vi "Write Data.vi"(8 "error in (no error)":errorcluster, 9 "Publication Time":timestamp, 10 "Value":variant, 11 "TerminalValueBinding In":refnum<class "TerminalValueBinding.lvclass">) -> (0 "error out":errorcluster, 3 "TerminalValueBinding Out":refnum<class "TerminalValueBinding.lvclass">)   [LabVIEW 2017, in "TerminalValueBinding.lvclass"]
doc: "<License>\nCopyright © 2017 Composed Systems, LLC | All rights reserved\nwww.composed.io\n\nAuthor: Ethan Stern <ethan.stern@composed.io>\n\nThis software is provided \"AS IS\" WITHOUT WARRANTIES, either express or implied, AND IS FOR EDUCATIONAL PURPOSES ONLY.\n</License>"
uses:
  <vilib>/gpm_packages/@cs/transport/Source/Concrete/TerminalValueBinding/TerminalValueBinding.lvclass
  <vilib>/gpm_packages/@cs/transport/Source/Concrete/TerminalValueBinding/TerminalValueBinding.lvclass/TerminalValueBinding.ctl
  <vilib>/Utility/error.llb/Error Cluster From Error Code.vi
  <vilib>/ErrorRing/Error Ring.xnode
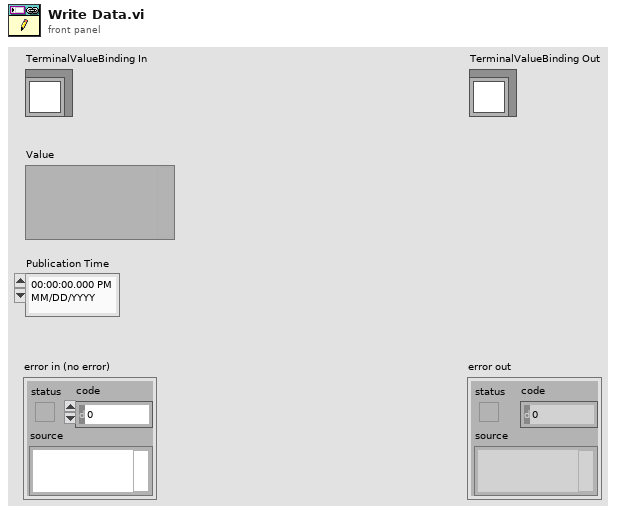
[diagram p1: front panel]
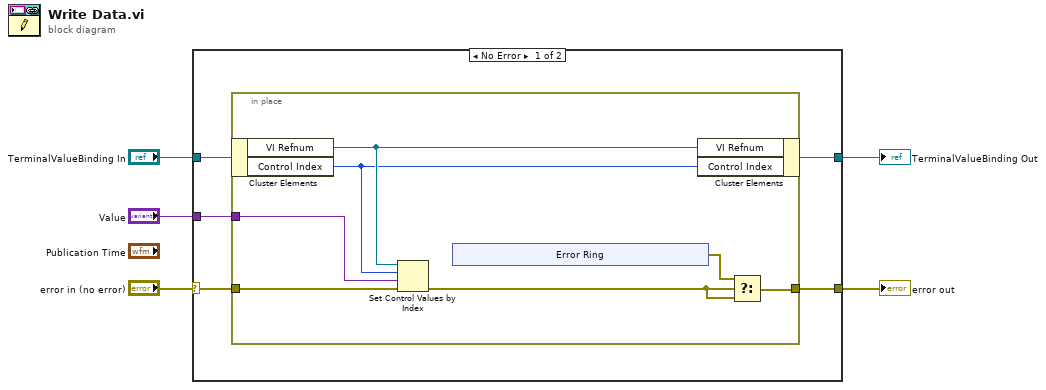
[diagram p0: block diagram]
diagram:
  n1 = case shown="No Error" "error in (no error)" {
    selector: "error in (no error)" -> [w10 w24]
    tunnel: "Value" -> [w9 _]
    tunnel: "TerminalValueBinding In" -> [w8 w23]
    tunnel: [w7 w23] -> w2
    tunnel: [w6 w24] -> w1
    frame No Error {
      n2 = in-place {
        in-place-border: w10 -> [w14]
        in-place-border: w9 -> [w15]
        in-place-border: [w11] -> w6
        n3 = in-place-cluster #1(w8) -> ("VI Refnum"=w17:refnum<vi>, "Control Index"=w16:i32)
        n4 = Set Control Values by Index(0:w17, 1:w16, 2:w15, 3:w14) -> (11:w13:errorcluster)
        n5 = xnode "Error Ring"() -> ("error out"=w12:errorcluster)
        n6 = in-place-cluster #1("VI Refnum"=w17, "Control Index"=w16) -> (w7:refnum<class "TerminalValueBinding.lvclass">)
        n7 = Select(t=w12, s=w13, f=w13) -> (s? t:f=w11:errorcluster)
      }
    }
    frame Error {
    }
  }
  "error out" <- w1
  "TerminalValueBinding Out" <- w2
